vi "SeqRun.vi"(2 "Error in":errorcluster, 3 "image size":cluster{"xpixels":i32, "ypixels":i32}, 4 "runs cluster":T2, 5 "Enabled pulse array 2":T3(array[cluster])) -> (0 "error out":errorcluster, 1 "step data":T1)   [LabVIEW 2017]
panel:
  out "last":i32
  out "first":u32
  out "DLL error code 2":u32
  out "kinetic series data":i32[][][][](array[numeric])
  out "DLL error code":u32
  out "times":u32[][](array[numeric])
  out "counts":cluster{u32[], u32[], u32[], u32[]}
  # "Inputs:"
  # "Outputs:"
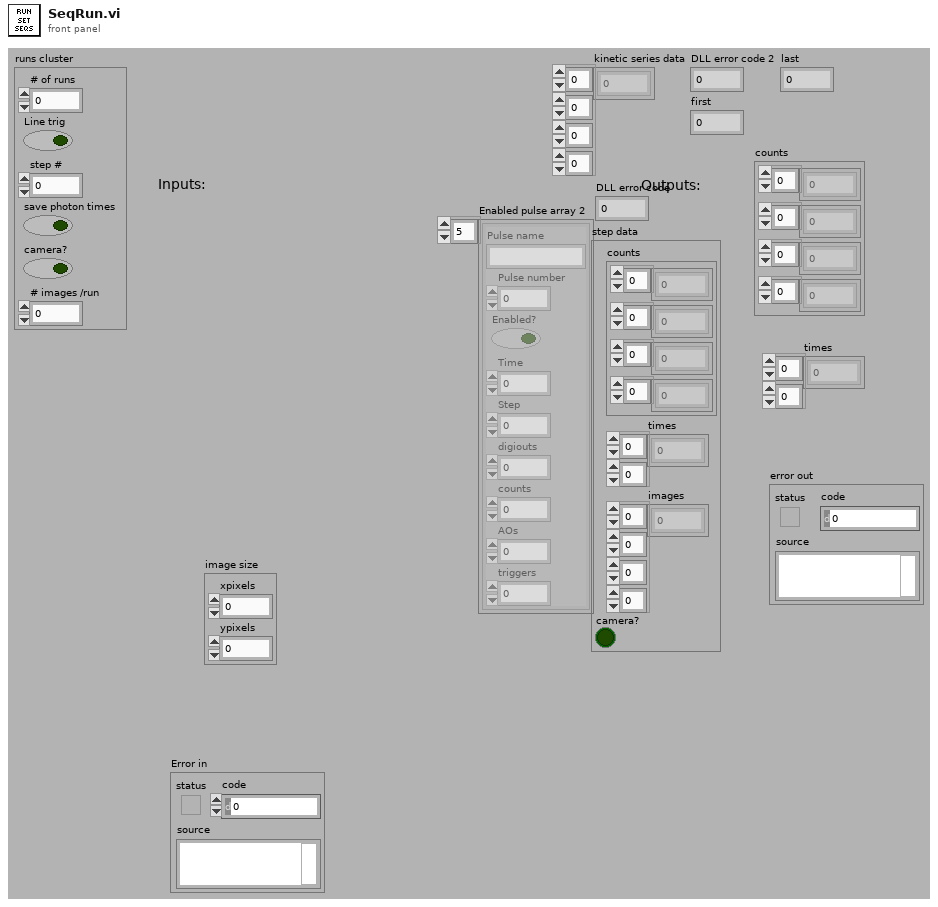
[diagram p1: front panel]
types:
  T1 = cluster{"counts":cluster{u32[], u32[], u32[], u32[]}, "times":u32[][], "images":i32[][][][], "camera?":bool}
  T2 = cluster{"# of runs":i32, "Line trig":bool, "step #":i32, "save photon times":bool, "camera?":bool, "# images /run":i8}
  T3 = cluster{"Pulse name":string, "Pulse number":i32, "Enabled?":bool, "Time":dbl, "Step":dbl, "digiouts":u64, "counts":u8, "AOs":u8, "triggers":u8}[]
  T4 = cluster{"Times":u32[], "Pulses":u64[], "Counts":u8[], "Triggers":u8[], "AOs":u8[], "# of runs":i32, "Line trig":bool, "save photon times":bool}
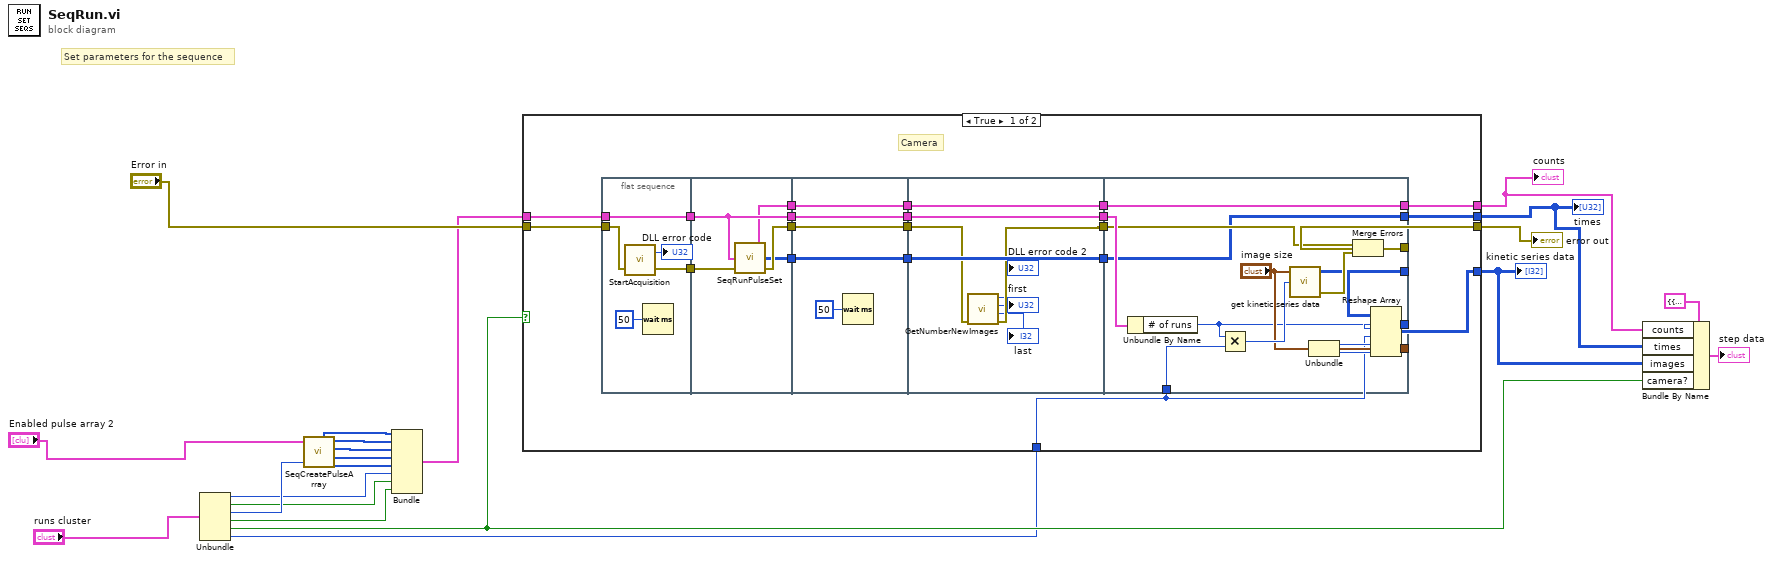
[diagram p0: block diagram]
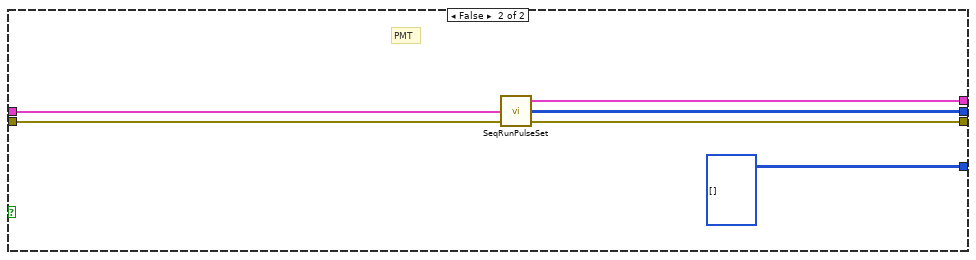
[diagram p2: hidden frame]
diagram:
  # "Set parameters for the sequence"
  n1 = Unbundle("runs cluster") -> ("# of runs"=w14:i32, "Line trig"=w10:bool, "step #"=w19:i32, "save photon times"=w9:bool, "camera?"=w6:bool, "# images /run"=w4:i8)
  n2 = call "SeqCreatePulseArray.vi"("Enabled pulse array 2"="Enabled pulse array 2", "step #"=w19) -> ("Pulses"=w12:u64[], "Times"=w15:u32[], "Counts"=w13:u8[], "Triggers"=w16:u8[], "AOs"=w17:u8[])  [unwired: 1 in, 1 out]
  n3 = Bundle("Times"=w15, "Pulses"=w12, "Counts"=w13, "Triggers"=w16, "AOs"=w17, "# of runs"=w14, "Line trig"=w10, "save photon times"=w9) -> (w11:T4)  [unwired: 1 in]
  n4 = case shown="True" w6 {
    tunnel: [w43 w87] -> w21
    tunnel: "Error in" -> [w47 w86]
    tunnel: w11 -> [w46 w85]
    tunnel: [w45 w84] -> w8
    tunnel: [w44 w83] -> w7
    tunnel: [w34 i32[][][][] [] ("kinetic series data")] -> w2
    tunnel: w4 -> [w36 _]
    frame True {
      # "Camera"
      n5 = flat-sequence {
        tunnel: w46 -> [w52]
        tunnel: w47 -> [w50]
        tunnel: [w49] -> w42
        tunnel: [w52] -> w41
        tunnel: w42 -> [w56]
        tunnel: [w55] -> w29
        tunnel: w41 -> [w57]
        tunnel: [w57] -> w27
        tunnel: [w54] -> w25
        tunnel: [w53] -> w23
        tunnel: w29 -> [w62]
        tunnel: [w62] -> w28
        tunnel: w27 -> [w61]
        tunnel: [w61] -> w26
        tunnel: w25 -> [w60]
        tunnel: [w60] -> w24
        tunnel: w23 -> [w59]
        tunnel: [w59] -> w22
        tunnel: w28 -> [w67]
        tunnel: [w66] -> w33
        tunnel: w26 -> [w70]
        tunnel: [w70] -> w32
        tunnel: w24 -> [w69]
        tunnel: [w69] -> w31
        tunnel: w22 -> [w68]
        tunnel: [w68] -> w30
        tunnel: [w76] -> w45
        tunnel: [w75] -> w44
        tunnel: w33 -> [w77]
        tunnel: w32 -> [w79]
        tunnel: [w80] -> w43
        tunnel: [w78] -> w39
        tunnel: w31 -> [w76]
        tunnel: w30 -> [w75]
        tunnel: w36 -> [w74]
        tunnel: ["image size"] -> w40
        tunnel: [w71] -> w35
        frame #0 {
          n6 = call <userlib>:"StartAcquisition.vi"("error in (no error)"=w50) -> ("error out"=w49:errorcluster, "DLL error code"=→"DLL error code":u32)  [unwired: 1 in]
          n7 = Wait (ms)(milliseconds to wait=u32 50) -> ()  [unwired: 1 out]
        }
        frame #1 {
          n8 = call "SeqRunPulseSet.vi"("error in"=w56, "Cluster"=w57) -> ("error out"=w55:errorcluster, "times"=w53:u32[][], "counts"=w54:cluster{u32[], u32[], u32[], u32[]})  [unwired: 1 in]
        }
        frame #2 {
          n9 = Wait (ms)(milliseconds to wait=u32 50) -> ()  [unwired: 1 out]
        }
        frame #3 {
          n10 = call <userlib>:"GetNumberNewImages.vi"("error in (no error)"=w67) -> ("error out"=w66:errorcluster, "last"=→"last":i32, "first"=→"first":u32, "DLL error code"=→"DLL error code 2":u32)  [unwired: 3 in]
        }
        frame #4 {
          n11 = Unbundle By Name(w79) -> ("# of runs"=w71:i32)
          n12 = Multiply(x=w71, y=w74) -> (x*y=w73:i32)
          n13 = call "get kinetic series data.vi"("# of kinetics"=w73, "image size"="image size") -> ("error out"=w81:errorcluster, "kinetic series data"=w78:i32[][][])  [unwired: 2 in]
          n14 = Merge Errors(w77, w81) -> (w80:errorcluster)
        }
      }
      n15 = Unbundle(w40) -> ("xpixels"=w37:i32, "ypixels"=w38:i32)
      n16 = Reshape Array(w39, w35, w36, w37, w38) -> (w34:i32[][][][])
    }
    frame False {
      # "PMT"
      n17 = call "SeqRunPulseSet.vi"("error in"=w86, "Cluster"=w85) -> ("error out"=w87:errorcluster, "times"=w83:u32[][], "counts"=w84:cluster{u32[], u32[], u32[], u32[]})  [unwired: 1 in]
    }
  }
  "error out" <- w21
  "counts" <- w8
  "times" <- w7
  "kinetic series data" <- w2
  n18 = Bundle By Name(cluster=T1 {"counts"={[], [], [], []}, "times"=[], "images"=[], "camera?"=FALSE} ("output cluster"), "counts"=w8, "times"=w7, "images"=w2, "camera?"=w6) -> (→"step data":T1)
